vi "run.vi"   [LabVIEW 2016, in "Test.lvrbt"]
uses:
  Test.lvrbt
  <vilib>/NXT/Block Support/NXT_InputPort.ctl
  <vilib>/NXT/Hardware/Plugins/Tetrix DC Motor/TetrixDCMotorAddress.ctl
  <vilib>/NXT/Hardware/Plugins/Tetrix 180 deg Servo/Tetrix180ServoAddress.ctl
  <vilib>/NXT/NXTIO Xnodes/NXTIONodeSubVIs/TETRIX IO Move Servos.vi
  <vilib>/NXT/Dual Mode Library/Waits/Wait_Num.vi
  <vilib>/NXT/NXTIO Xnodes/NXTIONodeSubVIs/TETRIX IO Move DC Motors.vi
  <vilib>/NXT/NXTIO Xnodes/NXTIONodeSubVIs/TETRIX IO Stop DC Motors.vi
  <vilib>/NXT/Dual Mode Library/Waits/Wait_EV3_Angle_Less.vi
  <vilib>/NXT/Dual Mode Library/Waits/Wait_EV3_Ultrasonic_Centimeter_Closer.vi
  <vilib>/NXT/Dual Mode Library/Waits/Wait_EV3_Angle_Greater.vi
  <vilib>/NXT/NXTIO Xnodes/AddressXNode/NXTIOAddress.xnode
  <vilib>/NXT/Subs/LVHSConnector.ctl
  <vilib>/NXT/NXTIO Xnodes/NXTIOXNode/NXTIO.xnode
  <vilib>/NXT/LegoClasses/BrickReference/BrickReference.lvclass
types:
  T1 = typedef "NXT_InputPort.ctl" = u32
  T2 = typedef "Tetrix180ServoAddress.ctl" = i32
  T3 = cluster{"Tetrix180Servo":T2, "Tetrix180Servo":T2, "Tetrix180Servo":T2}
  T4 = typedef "LVHSConnector.ctl" = refnum<class "BrickReference.lvclass">
  T5 = typedef "TetrixDCMotorAddress.ctl" = i32
  T6 = cluster{"Tetrix180Servo":T2, "Tetrix180Servo":T2}
diagram:
  w63 = T1 2 items=["Port 1", "Port 2", "Port 3", "Port 4"] ("Port (Port 1)")
  w105 = T1 2 items=["Port 1", "Port 2", "Port 3", "Port 4"] ("Port (Port 1)")
  w112 = T1 2 items=["Port 1", "Port 2", "Port 3", "Port 4"] ("Port (Port 1)")
  w148 = T1 1 items=["Port 1", "Port 2", "Port 3", "Port 4"] ("Port (Port 1)")
  w161 = T1 2 items=["Port 1", "Port 2", "Port 3", "Port 4"] ("Port (Port 1)")
  w171 = T1 2 items=["Port 1", "Port 2", "Port 3", "Port 4"] ("Port (Port 1)")
  w181 = T1 2 items=["Port 1", "Port 2", "Port 3", "Port 4"] ("Port (Port 1)")
  w238 = T1 1 items=["Port 1", "Port 2", "Port 3", "Port 4"] ("Port (Port 1)")
  # "Extra  :\n\nMove foward to aim"
  # "Extra  :\n\nMove foward to aim"
  # "PART 12 :\n\nBack to base"
  # "PART 11 :\n\nTurn angle to back to base"
  # "PART 10 :\n\nMove backward to back to base"
  # "PART 9 :\n\nMove back to the rack"
  # "PART 8 :\n\nSecond  aim to the goal and ready to release"
  # "PART 7 :\n\nMove backward to detect the second ball and ready to grab the ball"
  # "PART 6 :\n\nBack to the rack to grab second ball"
  # "PART 5 :\n\nTurn to aim the goal and ready to release the ball"
  # "PART 4 :\n\nGrab the ball and ready to aim"
  # "PART 3 :\n\nMove straight to detect the ball"
  # "PART 2 :\n\nTurn to the left -70 Deg"
  # "PART 1 :\n\nMove straight out from the base"
  n1 = xnode "Motors"() -> ("Motor"=w219:T3)
  n2 = xnode "Move Servos"("Position 3"=u8 0, "Position 2"=u8 0, "Position 1"=u8 131, "Motors"=w219) -> ("NXT/EV3"=w189:T4)  [unwired: 1 in]
  n3 = xnode "Motors"() -> ("Motor"=w253:cluster{"TetrixDCMotor":T5, "TetrixDCMotor":T5})
  n4 = call-poly <vilib>:"PolyWait.vi"("Time (1 sec)"=sgl 1.0, "NXT/EV3"=w189) -> ("NXT/EV3"=w215:T4)  [unwired: 2 in]
  n5 = xnode "Move Motors"("Power/Speed 2"=i8 80, "Power/Speed 1"=i8 80, "Motors"=w253, "NXT/EV3"=w215) -> ("NXT/EV3"=w250:T4)
  n6 = xnode "Motors"() -> ("Motor"=w188:cluster{"TetrixDCMotor":T5, "TetrixDCMotor":T5})
  n7 = call-poly <vilib>:"PolyWait.vi"("Time (1 sec)"=sgl 1.05, "NXT/EV3"=w250) -> ("NXT/EV3"=w187:T4)  [unwired: 2 in]
  n8 = xnode "Stop Motors"("Motors"=w188, "NXT/EV3"=w187) -> ("NXT/EV3"=w186:T4)
  n9 = xnode "Motors"() -> ("Motor"=w247:cluster{"TetrixDCMotor":T5, "TetrixDCMotor":T5})
  n10 = call-poly <vilib>:"PolyWait.vi"("Time (1 sec)"=sgl 1.7, "NXT/EV3"=w186) -> ("NXT/EV3"=w244:T4)  [unwired: 2 in]
  n11 = xnode "Move Motors"("Power/Speed 2"=i8 0, "Power/Speed 1"=i8 30, "Motors"=w247, "NXT/EV3"=w244) -> ("NXT/EV3"=w183:T4)
  n12 = call <vilib>:"EV3_Gyro_Reset.vi"("NXT/EV3"=w183, "Port (Port 1)"=w181) -> ("NXT/EV3"=w182:T4)  [unwired: 2 in]
  n13 = call-poly <vilib>:"PolyWait.vi"("Degrees (180)"=sgl -70.0, "NXT/EV3"=w182, "Port (Port 1)"=w181) -> ("NXT/EV3"=w180:T4)  [unwired: 1 in]
  n14 = xnode "Motors"() -> ("Motor"=w185:cluster{"TetrixDCMotor":T5, "TetrixDCMotor":T5})
  n15 = xnode "Stop Motors"("Motors"=w185, "NXT/EV3"=w180) -> ("NXT/EV3"=w184:T4)
  n16 = xnode "Motors"() -> ("Motor"=w243:cluster{"TetrixDCMotor":T5, "TetrixDCMotor":T5})
  n17 = call-poly <vilib>:"PolyWait.vi"("Time (1 sec)"=sgl 2.0, "NXT/EV3"=w184) -> ("NXT/EV3"=w209:T4)  [unwired: 2 in]
  n18 = xnode "Move Motors"("Power/Speed 2"=i8 18, "Power/Speed 1"=i8 18, "Motors"=w243, "NXT/EV3"=w209) -> ("NXT/EV3"=w240:T4)
  n19 = call-poly <vilib>:"PolyWait.vi"("Centimeters (40)"=sgl 15.0, "NXT/EV3"=w240, "Port (Port 1)"=w238) -> ("NXT/EV3"=w237:T4)  [unwired: 1 in]
  n20 = xnode "Motors"() -> ("Motor"=w236:cluster{"TetrixDCMotor":T5, "TetrixDCMotor":T5})
  n21 = xnode "Stop Motors"("Motors"=w236, "NXT/EV3"=w237) -> ("NXT/EV3"=w235:T4)
  n22 = xnode "Motors"() -> ("Motor"=w232:T6)
  n23 = call-poly <vilib>:"PolyWait.vi"("Time (1 sec)"=sgl 1.0, "NXT/EV3"=w235) -> ("NXT/EV3"=w233:T4)  [unwired: 2 in]
  n24 = xnode "Move Servos"("Position 2"=u8 0, "Position 1"=u8 0, "Motors"=w232, "NXT/EV3"=w233) -> ("NXT/EV3"=w207:T4)
  n25 = xnode "Motors"() -> ("Motor"=w213:T2)
  n26 = call-poly <vilib>:"PolyWait.vi"("Time (1 sec)"=sgl 1.2, "NXT/EV3"=w207) -> ("NXT/EV3"=w206:T4)  [unwired: 2 in]
  n27 = xnode "Move Servos"("Position 1"=u8 49, "Motors"=w213, "NXT/EV3"=w206) -> ("NXT/EV3"=w211:T4)
  n28 = xnode "Motors"() -> ("Motor"=w228:T2)
  n29 = call-poly <vilib>:"PolyWait.vi"("Time (1 sec)"=sgl 1.8, "NXT/EV3"=w211) -> ("NXT/EV3"=w226:T4)  [unwired: 2 in]
  n30 = xnode "Move Servos"("Position 1"=u8 131, "Motors"=w228, "NXT/EV3"=w226) -> ("NXT/EV3"=w225:T4)
  n31 = xnode "Motors"() -> ("Motor"=w222:T2)
  n32 = call-poly <vilib>:"PolyWait.vi"("Time (1 sec)"=sgl 1.8, "NXT/EV3"=w225) -> ("NXT/EV3"=w19:T4)  [unwired: 2 in]
  n33 = xnode "Motors"() -> ("Motor"=w24:cluster{"TetrixDCMotor":T5, "TetrixDCMotor":T5})
  n34 = xnode "Motors"() -> ("Motor"=w178:T2)
  n35 = xnode "Move Motors"("Power/Speed 2"=i8 30, "Power/Speed 1"=i8 30, "Motors"=w24, "NXT/EV3"=w19) -> ("NXT/EV3"=w22:T4)
  n36 = xnode "Motors"() -> ("Motor"=w18:cluster{"TetrixDCMotor":T5, "TetrixDCMotor":T5})
  n37 = call-poly <vilib>:"PolyWait.vi"("Time (1 sec)"=sgl 0.5, "NXT/EV3"=w22) -> ("NXT/EV3"=w17:T4)  [unwired: 2 in]
  n38 = xnode "Motors"() -> ("Motor"=w190:cluster{"TetrixDCMotor":T5, "TetrixDCMotor":T5})
  n39 = xnode "Stop Motors"("Motors"=w18, "NXT/EV3"=w17) -> ("NXT/EV3"=w15:T4)
  n40 = call-poly <vilib>:"PolyWait.vi"("Time (1 sec)"=sgl 0.5, "NXT/EV3"=w15) -> ("NXT/EV3"=w14:T4)  [unwired: 2 in]
  n41 = xnode "Move Servos"("Position 1"=u8 160, "Motors"=w222, "NXT/EV3"=w14) -> ("NXT/EV3"=w220:T4)
  n42 = call-poly <vilib>:"PolyWait.vi"("Time (1 sec)"=sgl 1.4, "NXT/EV3"=w220) -> ("NXT/EV3"=w176:T4)  [unwired: 2 in]
  n43 = xnode "Move Servos"("Position 1"=u8 5, "Motors"=w178, "NXT/EV3"=w176) -> ("NXT/EV3"=w174:T4)
  n44 = call-poly <vilib>:"PolyWait.vi"("Time (1 sec)"=sgl 1.4, "NXT/EV3"=w174) -> ("NXT/EV3"=w13:T4)  [unwired: 2 in]
  n45 = xnode "Move Motors"("Power/Speed 2"=i8 0, "Power/Speed 1"=i8 30, "Motors"=w190, "NXT/EV3"=w13) -> ("NXT/EV3"=w170:T4)
  n46 = call <vilib>:"EV3_Gyro_Reset.vi"("NXT/EV3"=w170, "Port (Port 1)"=w171) -> ("NXT/EV3"=w173:T4)  [unwired: 2 in]
  n47 = xnode "Motors"() -> ("Motor"=w169:cluster{"TetrixDCMotor":T5, "TetrixDCMotor":T5})
  n48 = call-poly <vilib>:"PolyWait.vi"("Degrees (180)"=sgl -1.5, "NXT/EV3"=w173, "Port (Port 1)"=w171) -> ("NXT/EV3"=w168:T4)  [unwired: 1 in]
  n49 = xnode "Stop Motors"("Motors"=w169, "NXT/EV3"=w168) -> ("NXT/EV3"=w166:T4)
  n50 = xnode "Motors"() -> ("Motor"=w205:T6)
  n51 = call-poly <vilib>:"PolyWait.vi"("Time (1 sec)"=sgl 1.0, "NXT/EV3"=w166) -> ("NXT/EV3"=w165:T4)  [unwired: 2 in]
  n52 = xnode "Move Servos"("Position 2"=u8 5, "Position 1"=u8 131, "Motors"=w205, "NXT/EV3"=w165) -> ("NXT/EV3"=w202:T4)
  n53 = xnode "Motors"() -> ("Motor"=w199:T2)
  n54 = call-poly <vilib>:"PolyWait.vi"("Time (1 sec)"=sgl 1.0, "NXT/EV3"=w202) -> ("NXT/EV3"=w200:T4)  [unwired: 2 in]
  n55 = xnode "Move Servos"("Position 1"=u8 80, "Motors"=w199, "NXT/EV3"=w200) -> ("NXT/EV3"=w196:T4)
  n56 = xnode "Motors"() -> ("Motor"=w194:T2)
  n57 = call-poly <vilib>:"PolyWait.vi"("Time (1 sec)"=sgl 1.5, "NXT/EV3"=w196) -> ("NXT/EV3"=w193:T4)  [unwired: 2 in]
  n58 = xnode "Move Servos"("Position 1"=u8 0, "Motors"=w194, "NXT/EV3"=w193) -> ("NXT/EV3"=w154:T4)
  n59 = xnode "Motors"() -> ("Motor"=w158:cluster{"TetrixDCMotor":T5, "TetrixDCMotor":T5})
  n60 = call-poly <vilib>:"PolyWait.vi"("Time (1 sec)"=sgl 1.5, "NXT/EV3"=w154) -> ("NXT/EV3"=w153:T4)  [unwired: 2 in]
  n61 = xnode "Move Motors"("Power/Speed 2"=i8 0, "Power/Speed 1"=i8 -30, "Motors"=w158, "NXT/EV3"=w153) -> ("NXT/EV3"=w162:T4)
  n62 = call <vilib>:"EV3_Gyro_Reset.vi"("NXT/EV3"=w162, "Port (Port 1)"=w161) -> ("NXT/EV3"=w159:T4)  [unwired: 2 in]
  n63 = xnode "Motors"() -> ("Motor"=w163:cluster{"TetrixDCMotor":T5, "TetrixDCMotor":T5})
  n64 = call-poly <vilib>:"PolyWait.vi"("Degrees (180)"=sgl 1.5, "NXT/EV3"=w159, "Port (Port 1)"=w161) -> ("NXT/EV3"=w164:T4)  [unwired: 1 in]
  n65 = xnode "Stop Motors"("Motors"=w163, "NXT/EV3"=w164) -> ("NXT/EV3"=w143:T4)
  n66 = xnode "Motors"() -> ("Motor"=w144:cluster{"TetrixDCMotor":T5, "TetrixDCMotor":T5})
  n67 = call-poly <vilib>:"PolyWait.vi"("Time (1 sec)"=sgl 2.0, "NXT/EV3"=w143) -> ("NXT/EV3"=w152:T4)  [unwired: 2 in]
  n68 = xnode "Move Motors"("Power/Speed 2"=i8 -25, "Power/Speed 1"=i8 -25, "Motors"=w144, "NXT/EV3"=w152) -> ("NXT/EV3"=w37:T4)
  n69 = xnode "Motors"() -> ("Motor"=w30:cluster{"TetrixDCMotor":T5, "TetrixDCMotor":T5})
  n70 = call-poly <vilib>:"PolyWait.vi"("Time (1 sec)"=sgl 0.8, "NXT/EV3"=w37) -> ("NXT/EV3"=w31:T4)  [unwired: 2 in]
  n71 = xnode "Stop Motors"("Motors"=w30, "NXT/EV3"=w31) -> ("NXT/EV3"=w27:T4)
  n72 = xnode "Motors"() -> ("Motor"=w33:cluster{"TetrixDCMotor":T5, "TetrixDCMotor":T5})
  n73 = call-poly <vilib>:"PolyWait.vi"("Time (1 sec)"=sgl 1.0, "NXT/EV3"=w27) -> ("NXT/EV3"=w28:T4)  [unwired: 2 in]
  n74 = xnode "Move Motors"("Power/Speed 2"=i8 18, "Power/Speed 1"=i8 18, "Motors"=w33, "NXT/EV3"=w28) -> ("NXT/EV3"=w32:T4)
  n75 = call-poly <vilib>:"PolyWait.vi"("Centimeters (40)"=sgl 15.0, "NXT/EV3"=w32, "Port (Port 1)"=w148) -> ("NXT/EV3"=w149:T4)  [unwired: 1 in]
  n76 = xnode "Motors"() -> ("Motor"=w150:cluster{"TetrixDCMotor":T5, "TetrixDCMotor":T5})
  n77 = xnode "Stop Motors"("Motors"=w150, "NXT/EV3"=w149) -> ("NXT/EV3"=w118:T4)
  n78 = xnode "Motors"() -> ("Motor"=w121:T6)
  n79 = call-poly <vilib>:"PolyWait.vi"("Time (1 sec)"=sgl 1.0, "NXT/EV3"=w118) -> ("NXT/EV3"=w120:T4)  [unwired: 2 in]
  n80 = xnode "Move Servos"("Position 2"=u8 0, "Position 1"=u8 0, "Motors"=w121, "NXT/EV3"=w120) -> ("NXT/EV3"=w138:T4)
  n81 = xnode "Motors"() -> ("Motor"=w134:T2)
  n82 = call-poly <vilib>:"PolyWait.vi"("Time (1 sec)"=sgl 1.2, "NXT/EV3"=w138) -> ("NXT/EV3"=w139:T4)  [unwired: 2 in]
  n83 = xnode "Move Servos"("Position 1"=u8 49, "Motors"=w134, "NXT/EV3"=w139) -> ("NXT/EV3"=w136:T4)
  n84 = xnode "Motors"() -> ("Motor"=w125:T2)
  n85 = call-poly <vilib>:"PolyWait.vi"("Time (1 sec)"=sgl 1.8, "NXT/EV3"=w136) -> ("NXT/EV3"=w127:T4)  [unwired: 2 in]
  n86 = xnode "Move Servos"("Position 1"=u8 131, "Motors"=w125, "NXT/EV3"=w127) -> ("NXT/EV3"=w128:T4)
  n87 = xnode "Motors"() -> ("Motor"=w131:T2)
  n88 = xnode "Motors"() -> ("Motor"=w10:cluster{"TetrixDCMotor":T5, "TetrixDCMotor":T5})
  n89 = call-poly <vilib>:"PolyWait.vi"("Time (1 sec)"=sgl 1.8, "NXT/EV3"=w128) -> ("NXT/EV3"=w3:T4)  [unwired: 2 in]
  n90 = xnode "Move Motors"("Power/Speed 2"=i8 30, "Power/Speed 1"=i8 30, "Motors"=w10, "NXT/EV3"=w3) -> ("NXT/EV3"=w8:T4)
  n91 = xnode "Motors"() -> ("Motor"=w7:cluster{"TetrixDCMotor":T5, "TetrixDCMotor":T5})
  n92 = xnode "Motors"() -> ("Motor"=w140:T2)
  n93 = call-poly <vilib>:"PolyWait.vi"("Time (1 sec)"=sgl 0.5, "NXT/EV3"=w8) -> ("NXT/EV3"=w6:T4)  [unwired: 2 in]
  n94 = xnode "Stop Motors"("Motors"=w7, "NXT/EV3"=w6) -> ("NXT/EV3"=w4:T4)
  n95 = xnode "Motors"() -> ("Motor"=w115:cluster{"TetrixDCMotor":T5, "TetrixDCMotor":T5})
  n96 = call-poly <vilib>:"PolyWait.vi"("Time (1 sec)"=sgl 0.5, "NXT/EV3"=w4) -> ("NXT/EV3"=w2:T4)  [unwired: 2 in]
  n97 = xnode "Move Servos"("Position 1"=u8 160, "Motors"=w131, "NXT/EV3"=w2) -> ("NXT/EV3"=w133:T4)
  n98 = call-poly <vilib>:"PolyWait.vi"("Time (1 sec)"=sgl 1.4, "NXT/EV3"=w133) -> ("NXT/EV3"=w142:T4)  [unwired: 2 in]
  n99 = xnode "Move Servos"("Position 1"=u8 5, "Motors"=w140, "NXT/EV3"=w142) -> ("NXT/EV3"=w20:T4)
  n100 = call-poly <vilib>:"PolyWait.vi"("Time (1 sec)"=sgl 1.4, "NXT/EV3"=w20) -> ("NXT/EV3"=w1:T4)  [unwired: 2 in]
  n101 = xnode "Move Motors"("Power/Speed 2"=i8 0, "Power/Speed 1"=i8 30, "Motors"=w115, "NXT/EV3"=w1) -> ("NXT/EV3"=w111:T4)
  n102 = call <vilib>:"EV3_Gyro_Reset.vi"("NXT/EV3"=w111, "Port (Port 1)"=w112) -> ("NXT/EV3"=w114:T4)  [unwired: 2 in]
  n103 = xnode "Motors"() -> ("Motor"=w110:cluster{"TetrixDCMotor":T5, "TetrixDCMotor":T5})
  n104 = call-poly <vilib>:"PolyWait.vi"("Degrees (180)"=sgl -4.0, "NXT/EV3"=w114, "Port (Port 1)"=w112) -> ("NXT/EV3"=w109:T4)  [unwired: 1 in]
  n105 = xnode "Stop Motors"("Motors"=w110, "NXT/EV3"=w109) -> ("NXT/EV3"=w71:T4)
  n106 = xnode "Motors"() -> ("Motor"=w75:T6)
  n107 = call-poly <vilib>:"PolyWait.vi"("Time (1 sec)"=sgl 1.0, "NXT/EV3"=w71) -> ("NXT/EV3"=w89:T4)  [unwired: 2 in]
  n108 = xnode "Move Servos"("Position 2"=u8 5, "Position 1"=u8 131, "Motors"=w75, "NXT/EV3"=w89) -> ("NXT/EV3"=w78:T4)
  n109 = xnode "Motors"() -> ("Motor"=w81:T2)
  n110 = call-poly <vilib>:"PolyWait.vi"("Time (1 sec)"=sgl 2.0, "NXT/EV3"=w78) -> ("NXT/EV3"=w80:T4)  [unwired: 2 in]
  n111 = xnode "Move Servos"("Position 1"=u8 80, "Motors"=w81, "NXT/EV3"=w80) -> ("NXT/EV3"=w84:T4)
  n112 = xnode "Motors"() -> ("Motor"=w86:T2)
  n113 = call-poly <vilib>:"PolyWait.vi"("Time (1 sec)"=sgl 1.5, "NXT/EV3"=w84) -> ("NXT/EV3"=w87:T4)  [unwired: 2 in]
  n114 = xnode "Move Servos"("Position 1"=u8 0, "Motors"=w86, "NXT/EV3"=w87) -> ("NXT/EV3"=w73:T4)
  n115 = xnode "Motors"() -> ("Motor"=w102:cluster{"TetrixDCMotor":T5, "TetrixDCMotor":T5})
  n116 = call-poly <vilib>:"PolyWait.vi"("Time (1 sec)"=sgl 1.5, "NXT/EV3"=w73) -> ("NXT/EV3"=w72:T4)  [unwired: 2 in]
  n117 = xnode "Move Motors"("Power/Speed 2"=i8 0, "Power/Speed 1"=i8 -30, "Motors"=w102, "NXT/EV3"=w72) -> ("NXT/EV3"=w106:T4)
  n118 = call <vilib>:"EV3_Gyro_Reset.vi"("NXT/EV3"=w106, "Port (Port 1)"=w105) -> ("NXT/EV3"=w103:T4)  [unwired: 2 in]
  n119 = xnode "Motors"() -> ("Motor"=w107:cluster{"TetrixDCMotor":T5, "TetrixDCMotor":T5})
  n120 = call-poly <vilib>:"PolyWait.vi"("Degrees (180)"=sgl 4.0, "NXT/EV3"=w103, "Port (Port 1)"=w105) -> ("NXT/EV3"=w108:T4)  [unwired: 1 in]
  n121 = xnode "Stop Motors"("Motors"=w107, "NXT/EV3"=w108) -> ("NXT/EV3"=w98:T4)
  n122 = xnode "Motors"() -> ("Motor"=w95:cluster{"TetrixDCMotor":T5, "TetrixDCMotor":T5})
  n123 = call-poly <vilib>:"PolyWait.vi"("Time (1 sec)"=sgl 1.8, "NXT/EV3"=w98) -> ("NXT/EV3"=w94:T4)  [unwired: 2 in]
  n124 = xnode "Move Motors"("Power/Speed 2"=i8 -80, "Power/Speed 1"=i8 -80, "Motors"=w95, "NXT/EV3"=w94) -> ("NXT/EV3"=w92:T4)
  n125 = xnode "Motors"() -> ("Motor"=w91:cluster{"TetrixDCMotor":T5, "TetrixDCMotor":T5})
  n126 = call-poly <vilib>:"PolyWait.vi"("Time (1 sec)"=sgl 1.0, "NXT/EV3"=w92) -> ("NXT/EV3"=w90:T4)  [unwired: 2 in]
  n127 = xnode "Stop Motors"("Motors"=w91, "NXT/EV3"=w90) -> ("NXT/EV3"=w70:T4)
  n128 = xnode "Motors"() -> ("Motor"=w66:cluster{"TetrixDCMotor":T5, "TetrixDCMotor":T5})
  n129 = call-poly <vilib>:"PolyWait.vi"("Time (1 sec)"=sgl 1.0, "NXT/EV3"=w70) -> ("NXT/EV3"=w59:T4)  [unwired: 2 in]
  n130 = xnode "Move Motors"("Power/Speed 2"=i8 0, "Power/Speed 1"=i8 -30, "Motors"=w66, "NXT/EV3"=w59) -> ("NXT/EV3"=w62:T4)
  n131 = call <vilib>:"EV3_Gyro_Reset.vi"("NXT/EV3"=w62, "Port (Port 1)"=w63) -> ("NXT/EV3"=w65:T4)  [unwired: 2 in]
  n132 = xnode "Motors"() -> ("Motor"=w61:cluster{"TetrixDCMotor":T5, "TetrixDCMotor":T5})
  n133 = call-poly <vilib>:"PolyWait.vi"("Degrees (180)"=sgl 70.0, "NXT/EV3"=w65, "Port (Port 1)"=w63) -> ("NXT/EV3"=w60:T4)  [unwired: 1 in]
  n134 = xnode "Stop Motors"("Motors"=w61, "NXT/EV3"=w60) -> ("NXT/EV3"=w57:T4)
  n135 = xnode "Motors"() -> ("Motor"=w52:cluster{"TetrixDCMotor":T5, "TetrixDCMotor":T5})
  n136 = call-poly <vilib>:"PolyWait.vi"("Time (1 sec)"=sgl 1.0, "NXT/EV3"=w57) -> ("NXT/EV3"=w49:T4)  [unwired: 2 in]
  n137 = xnode "Move Motors"("Power/Speed 2"=i8 -80, "Power/Speed 1"=i8 -80, "Motors"=w52, "NXT/EV3"=w49) -> ("NXT/EV3"=w54:T4)
  n138 = xnode "Motors"() -> ("Motor"=w55:cluster{"TetrixDCMotor":T5, "TetrixDCMotor":T5})
  n139 = call-poly <vilib>:"PolyWait.vi"("Time (1 sec)"=sgl 0.9, "NXT/EV3"=w54) -> ("NXT/EV3"=w56:T4)  [unwired: 2 in]
  n140 = xnode "Stop Motors"("Motors"=w55, "NXT/EV3"=w56) -> ("NXT/EV3"=w48:T4)
  n141 = xnode "Motors"() -> ("Motor"=w45:T6)
  n142 = call-poly <vilib>:"PolyWait.vi"("Time (1 sec)"=sgl 1.0, "NXT/EV3"=w48) -> ("NXT/EV3"=w46:T4)  [unwired: 2 in]
  n143 = xnode "Move Servos"("Position 2"=u8 0, "Position 1"=u8 5, "Motors"=w45, "NXT/EV3"=w46) -> ("NXT/EV3"=w41:T4)
  n144 = xnode "Motors"() -> ("Motor"=w39:T2)
  n145 = call-poly <vilib>:"PolyWait.vi"("Time (1 sec)"=sgl 0.5, "NXT/EV3"=w41) -> ("NXT/EV3"=w40:T4)  [unwired: 2 in]
  n146 = xnode "Move Servos"("Position 1"=u8 0, "Motors"=w39, "NXT/EV3"=w40) -> ()  [unwired: 1 out]
